vi "Read Page Button Properties.vi"(8 "Error In":errorcluster, 11 "Custom Device Page .NET Ref In":refnum<k24>) -> (0 "Error Out":errorcluster, 2 "All Button Properties":T1[](array[typedef]), 3 "Custom Device Page .NET Ref Out":refnum<k24>)   [LabVIEW 2019, in "VeriStand Custom Device XML Parser.lvlib"]
doc: "Reads and returns the properties of all buttons for the page"
uses:
  VeriStand Custom Device XML Parser.lvlib
  XML Controls/Button Properties.ctl
  XML Controls/Path Cluster.ctl
  XML Controls/Button Type.ctl
  XML Controls/Dependency Properties.ctl
  NationalInstruments.VeriStand.XMLReader
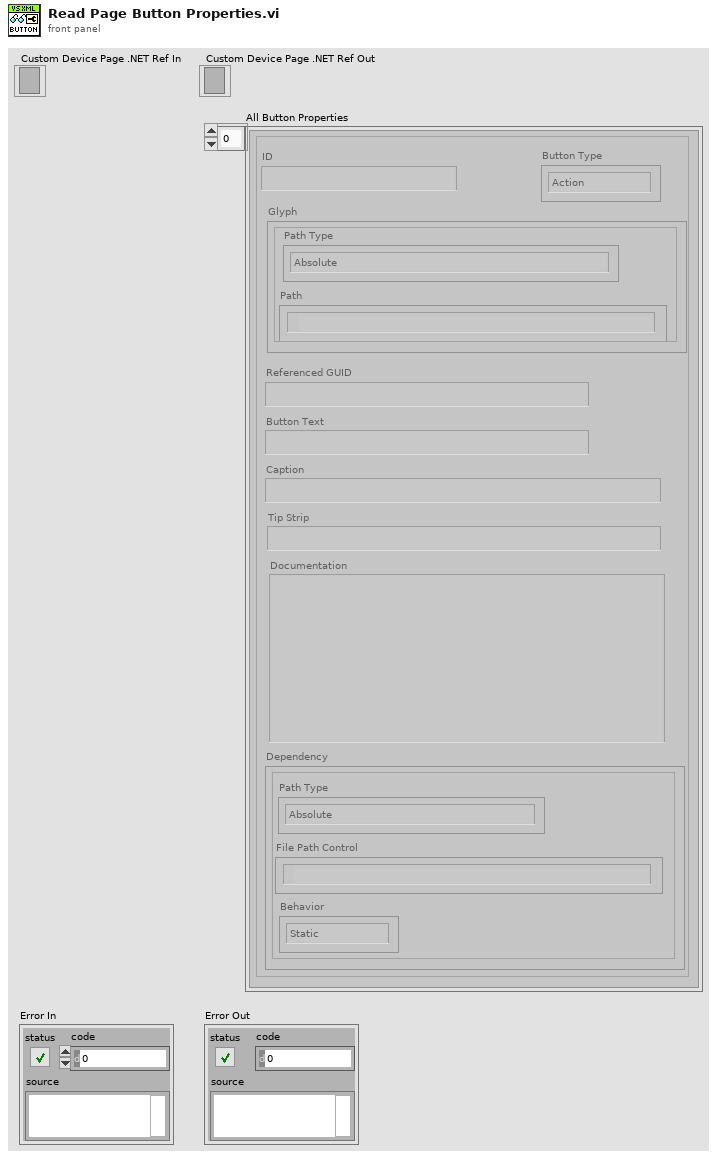
[diagram p1: front panel]
types:
  T1 = typedef "VeriStand Custom Device XML Parser.lvlib/Button Properties.ctl" = cluster{"ID":string, "Glyph":T2, "Button Type":T3, "Referenced GUID":string, "Button Text":string, "Caption":string, "Tip Strip":string, "Documentation":string, "Dependency":T4}
  T2 = typedef "VeriStand Custom Device XML Parser.lvlib/Path Cluster.ctl" = cluster{"Path":path, "Path Type":enum16{"Absolute", "To Base", "To Common Doc Dir", "To Application Data Dir"}}
  T3 = typedef "VeriStand Custom Device XML Parser.lvlib/Button Type.ctl" = enum16{"Action", "Dialog", "Page", "Notification", "Separator"}
  T4 = typedef "VeriStand Custom Device XML Parser.lvlib/Dependency Properties.ctl" = cluster{"File Path Control":path, "Path Type":enum16{"Absolute", "To Base", "To Common Doc Dir", "To Application Data Dir"}, "Behavior":enum16{"Static", "Dynamic"}}
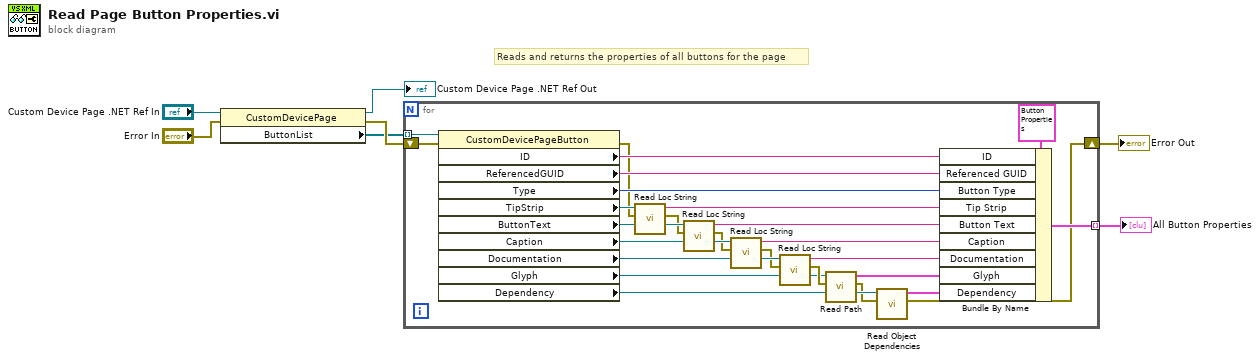
[diagram p0: block diagram]
diagram:
  # "Reads and returns the properties of all buttons for the page"
  n1 = property class="CustomDevicePage"(reference="Custom Device Page .NET Ref In", error in="Error In") -> (reference out=→"Custom Device Page .NET Ref Out":refnum<k24>, error out=w4:errorcluster, "ButtonList"=w3:refnum<k24>[])
  n2 = for {
    tunnel: w3 -> [w32] mode=indexing
    shift-right: [w8] -> w6
    shift-left: w4 -> [w33]
    tunnel: [w11] -> w7 mode=indexing
    n3 = property class="CustomDevicePageButton"(reference=w32, error in=w33) -> (error out=w26:errorcluster, "ID"=w30:string, "ReferencedGUID"=w29:string, "Type"=w28:i32, "TipStrip"=w27:refnum<k24>, "ButtonText"=w24:refnum<k24>, "Caption"=w21:refnum<k24>, "Documentation"=w20:refnum<k24>, "Glyph"=w16:refnum<k24>, "Dependency"=w12:refnum<k24>)  [unwired: 1 out]
    n4 = call "Read Loc String.vi"("Error In"=w26, "Loc String .NET Ref"=w27) -> ("Error Out"=w23:errorcluster, "English"=w25:string)  [unwired: 7 in, 1 out]
    n5 = call "Read Loc String.vi"("Error In"=w23, "Loc String .NET Ref"=w24) -> ("Error Out"=w19:errorcluster, "English"=w22:string)  [unwired: 7 in, 1 out]
    n6 = call "Read Loc String.vi"("Error In"=w19, "Loc String .NET Ref"=w21) -> ("Error Out"=w18:errorcluster, "English"=w15:string)  [unwired: 7 in, 1 out]
    n7 = call "Read Loc String.vi"("Error In"=w18, "Loc String .NET Ref"=w20) -> ("Error Out"=w17:errorcluster, "English"=w14:string)  [unwired: 7 in, 1 out]
    n8 = call "Read Path.vi"("Error In"=w17, "Path .NET Ref"=w16) -> ("Error Out"=w9:errorcluster, "Path Properties"=w13:T2)  [unwired: 8 in]
    n9 = call "Read Object Dependencies.vi"("Error In"=w9, "Dependency .NET Ref In"=w12) -> ("Error Out"=w8:errorcluster, "Dependency Properties"=w10:T4)  [unwired: 8 in]
    n10 = Bundle By Name(cluster=T1 {"ID"="", "Glyph"={"Path"=path "", "Path Type"=enum."Absolute"}, "Button Type"=enum."Action", "Referenced GUID"="", "Button Text"="", "Caption"="", "Tip Strip"="", "Documentation"="", "Dependency"={"File Path Control"=path "", "Path Type"=enum."Absolute", "Behavior"=enum."Static"}} ("Button"), "ID"=w30, "Referenced GUID"=w29, "Button Type"=w28, "Tip Strip"=w25, "Button Text"=w22, "Caption"=w15, "Documentation"=w14, "Glyph"=w13, "Dependency"=w10) -> (w11:T1)
  }
  "All Button Properties" <- w7
  "Error Out" <- w6
